vi "test-cubic-spline-00.vi"() -> (3 "Test Passed":bool)   [LabVIEW 2019]
uses:
  <vilib>/Rock Robotics/WPI/ThirdParty/JAS_Junk/TrajLib/POSEwCURVATURE.ctl
  <vilib>/Rock Robotics/WPI/ThirdParty/JAS_Junk/TrajLib/POSE2D.ctl
  <vilib>/Rock Robotics/WPI/ThirdParty/JAS_Junk/TrajLib/TRANSLATION2D.ctl
  <vilib>/Rock Robotics/WPI/ThirdParty/JAS_Junk/TrajLib/ROTATION2D.ctl
  <vilib>/Rock Robotics/WPI/ThirdParty/JAS_Junk/TrajLib/Rotation_CreateAngle.vi
  <vilib>/Rock Robotics/WPI/ThirdParty/JAS_Junk/TrajLib/Translation_Create.vi
  <vilib>/Rock Robotics/WPI/ThirdParty/JAS_Junk/TrajLib/Util_CalcDist.vi
  <vilib>/Rock Robotics/WPI/ThirdParty/JAS_Junk/TrajLib/Trajectory_Library.lvlib
panel:
  out "XY Graph":cluster{dbl[], dbl[]}(graph)
  out "All Interior \nwayPoints\nFound (True)":bool
  out "end rot = 0":dbl
  out "end y = 0":dbl
  out "end x = 0":dbl
  out "start rot = 0":dbl
  out "start y = 0":dbl
  out "start x = 0":dbl
  out "max dtheta < 0.0872":dbl
  out "max dy < 0.00127":dbl
  out "max dx  < 0.127":dbl
  out "Overall Error":errorcluster
  out "Elements":i32
  out "Create Spline Error":errorcluster
  out "SplinePoses\nWCurve":T1[](array[typedef]) {"POSE"."ROTATION"."SIN" format="%13.4f"; "POSE"."ROTATION"."COS" format="%13.4f"; "POSE"."ROTATION"."VALUE" format="%13.4f"; "POSE"."TRANSLATION"."Y" format="%14.3f"; "POSE"."TRANSLATION"."X" format="%14.3f"}
  out "Elapsed Time":dbl
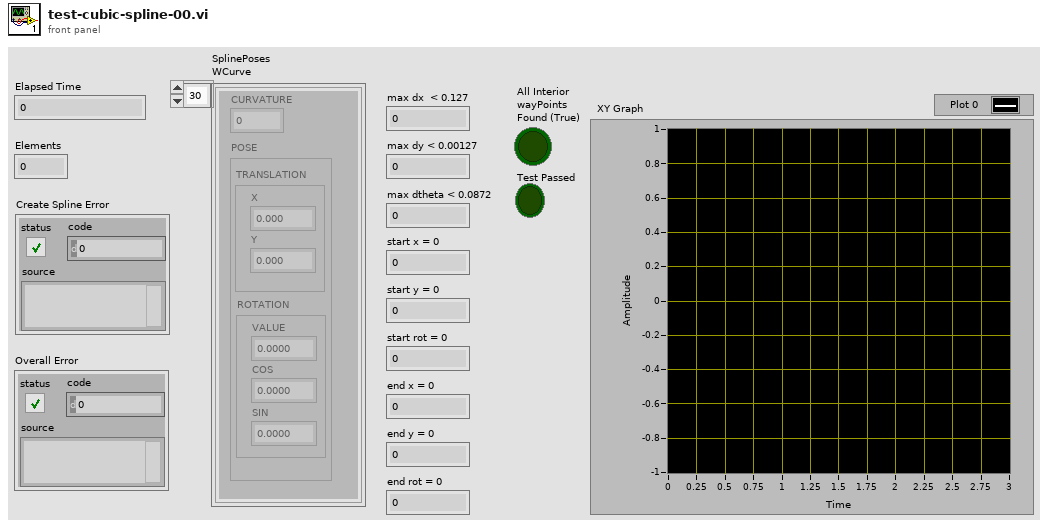
[diagram p1: front panel]
types:
  T1 = typedef "Trajectory_Library.lvlib/POSEwCURVATURE.ctl" = cluster{"CURVATURE":dbl, "POSE":T2}
  T2 = typedef "Trajectory_Library.lvlib/POSE2D.ctl" = cluster{"TRANSLATION":T3, "ROTATION":T4}
  T3 = typedef "Trajectory_Library.lvlib/TRANSLATION2D.ctl" = cluster{"X":dbl, "Y":dbl}
  T4 = typedef "Trajectory_Library.lvlib/ROTATION2D.ctl" = cluster{"VALUE":dbl, "COS":dbl, "SIN":dbl}
  T5 = typedef "Trajectory_Library.lvlib/SPLINE_CTRL_VECTOR.ctl" = cluster{"Xs":dbl[], "Ys":dbl[]}
  T6 = typedef "Trajectory_Library.lvlib/SPLINE.ctl" = cluster{"Degree":i32, "Coefficients":T7}
  T7 = typedef "NI_Matrix.lvlib/RealMatrix.ctl" = dbl[][]
  T8 = typedef "Trajectory_Library.lvlib/TWIST2D.ctl" = cluster{"dX":dbl, "dY":dbl, "dTHETA":dbl}
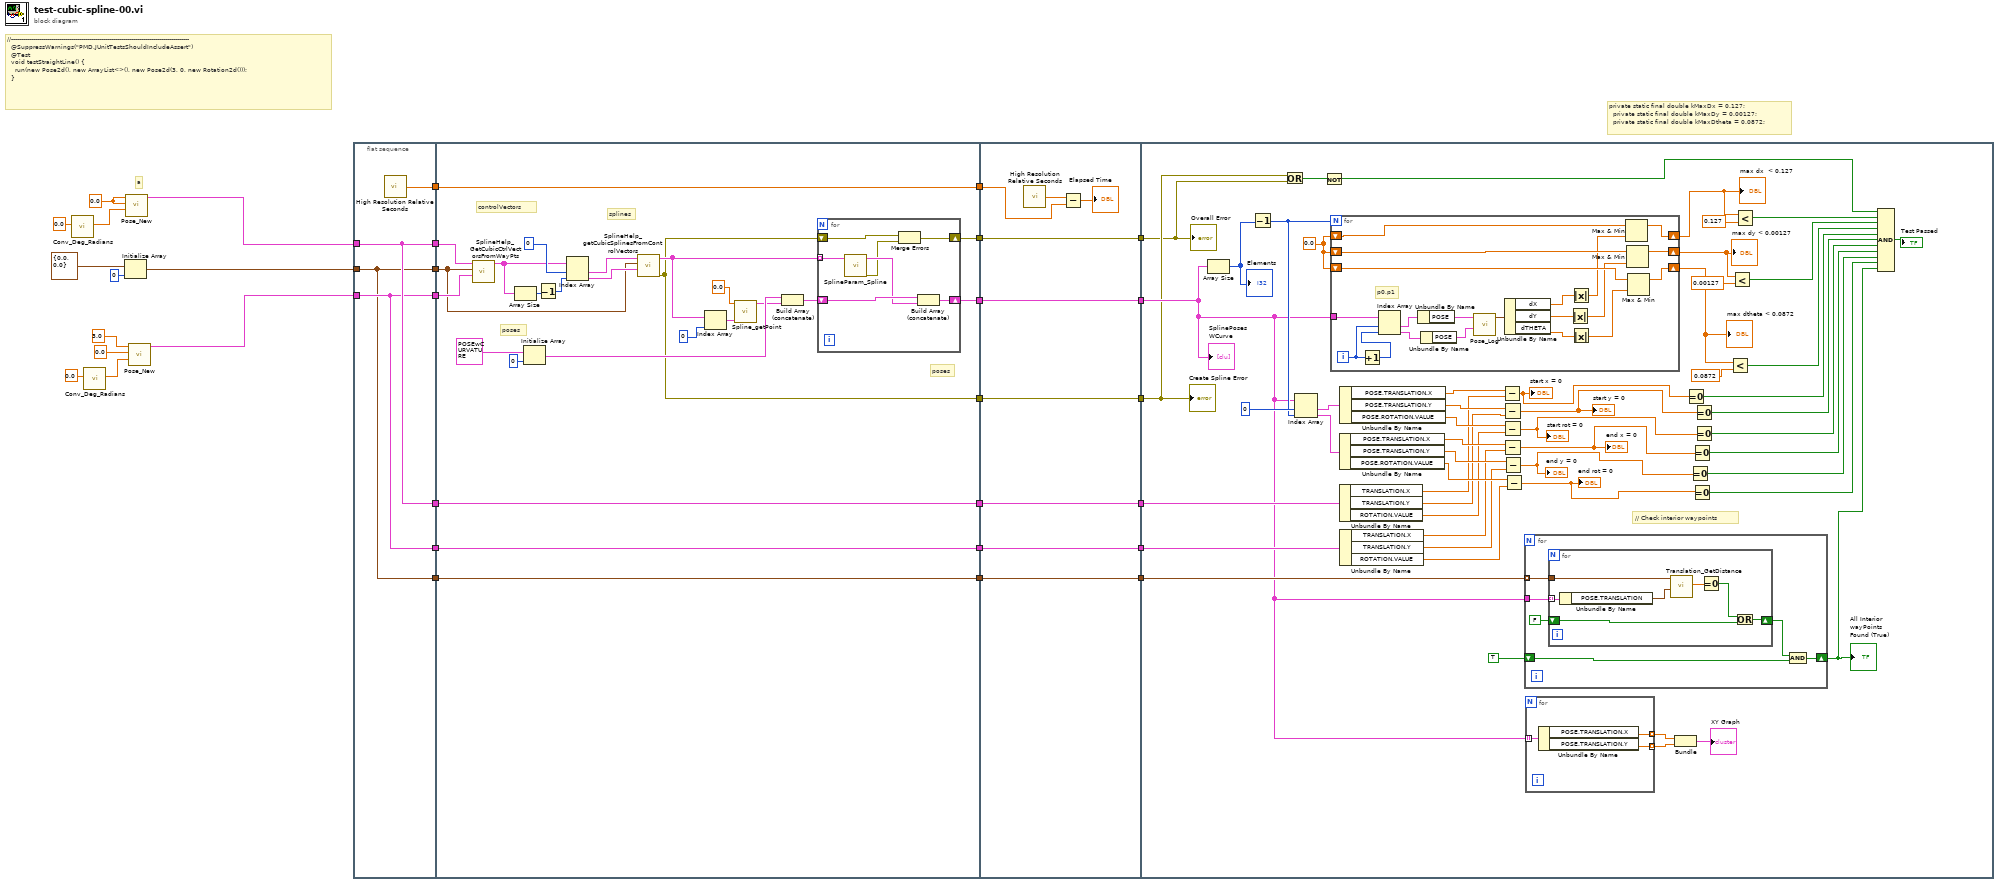
[diagram p0: block diagram]
diagram:
  w8 = 0.0 ("X")
  # "private static final double kMaxDx = 0.127;\n  private static final double kMaxDy = 0.00127;\n  private static final double kMaxDtheta = 0.0872;"
  # "a"
  # "//-----------------------------------------------------------------------------------------\n  @SuppressWarnings(\"PMD.JUnitTestsShouldIncludeAssert\")\n  @Test\n  void testStraightLine() {\n    run(new Pose2d(), new ArrayList<>(), new Pose2d(3, 0, new Rotation2d()));\n  }"
  n1 = call <vilib>:"Conv_Deg_Radians.vi"("Degress"=0.0) -> ("Radians"=w7:dbl)  [unwired: 10 in]
  n2 = call <vilib>:"Conv_Deg_Radians.vi"("Degress"=0.0) -> ("Radians"=w4:dbl)  [unwired: 10 in]
  n3 = Initialize Array(T3 {"X"=0.0, "Y"=0.0} ("TRANSLATION"), 0 ("dimension size")) -> (w1:T3[])
  n4 = call <vilib>:"Pose_New.vi"("Heading"=w7, "Y"=w8, "X"=w8) -> ("out POSe"=w30:T2)  [unwired: 8 in]
  n5 = call <vilib>:"Pose_New.vi"("Heading"=w4, "Y"=0.0, "X"=3.0) -> ("out POSe"=w27:T2)  [unwired: 8 in]
  n6 = flat-sequence {
    tunnel: w30 -> [w35]
    tunnel: [w35] -> w29
    tunnel: w1 -> [w33]
    tunnel: [w33] -> w28
    tunnel: w27 -> [w34]
    tunnel: [w34] -> w26
    tunnel: [w36] -> w25
    tunnel: [w35] -> w17
    tunnel: [w34] -> w14
    tunnel: [w33] -> w9
    tunnel: w29 -> [w61]
    tunnel: w28 -> [w53]
    tunnel: w26 -> [w60]
    tunnel: [w52] -> w24
    tunnel: w25 -> [w52]
    tunnel: [w42] -> w23
    tunnel: [w41] -> w21
    tunnel: [w40] -> w19
    tunnel: w17 -> [w39]
    tunnel: [w39] -> w16
    tunnel: w14 -> [w38]
    tunnel: [w38] -> w13
    tunnel: [w37] -> w10
    tunnel: w9 -> [w37]
    tunnel: w24 -> [w77]
    tunnel: w23 -> [w76]
    tunnel: [w76] -> w22
    tunnel: w21 -> [w75]
    tunnel: [w75] -> w20
    tunnel: w19 -> [w74]
    tunnel: [w74] -> w18
    tunnel: w16 -> [w71]
    tunnel: [w71] -> w15
    tunnel: w13 -> [w70]
    tunnel: [w70] -> w12
    tunnel: [w69] -> w11
    tunnel: w10 -> [w69]
    tunnel: w22 -> [w105]
    tunnel: w20 -> [w80]
    tunnel: w18 -> [w79]
    tunnel: w15 -> [w128]
    tunnel: w12 -> [w127]
    tunnel: w11 -> [w110]
    frame #0 {
      n7 = call <vilib>:"High Resolution Relative Seconds.vi"() -> ("relative seconds"=w36:dbl)
    }
    frame #1 {
      # "poses"
      # "poses"
      # "splines"
      # "controlVectors"
      n8 = call <vilib>:"SplineHelp_GetCubicCtrlVectorsFromWayPts.vi"("Enging POSE"=w60, "Interior WAYPOINTS"=w53, "Starting POSE"=w61) -> ("SplineControlVectors"=w57:T5[])  [unwired: 8 in]
      n9 = Array Size(array=w57) -> (size(s)=w58:i32)
      n10 = Initialize Array(T1 {"CURVATURE"=0.0, "POSE"={"TRANSLATION"={"X"=0.0, "Y"=0.0}, "ROTATION"={"VALUE"=0.0, "COS"=1.0, "SIN"=0.0}}} ("POSEwCURVATURE"), 0 ("dimension size")) -> (w46:T1[])
      n11 = Decrement(x=w58) -> (x-1=w56:i32)
      n12 = Index Array(array=w57, index #1=0 ("index"), index #2=w56) -> (element #1=w55:T5, element #2=w54:T5)
      n13 = call <vilib>:"SplineHelp_getCubicSplinesFromControlVectors.vi"("endCtrlVector"=w54, "InternalWaypoints"=w53, "startCtrlVector"=w55) -> ("error out"=w41:errorcluster, "splines"=w43:T6[])  [unwired: 3 in, 4 out]
      n14 = Index Array(array=w43, index=0) -> (element=w48:T6)
      n15 = call <vilib>:"Spline_getPoint.vi"("inputSPLINE"=w48, "Time"=0.0) -> ("POSEwCURVATURE"=w45:T1)  [unwired: 9 in]
      n16 = Build Array (concatenate)(w46, w45) -> (w44:T1[])
      n17 = for {
        shift-right: [w65] -> w42
        shift-left: w44 -> [w67]
        tunnel: w43 -> [w68] mode=indexing
        shift-right: [w63] -> w40
        shift-left: w41 -> [w64]
        n18 = call <vilib>:"SplineParam_Spline.vi"("inputSPLINE"=w68) -> ("error out"=w62:errorcluster, "outputPOSEwCURVATURE"=w66:T1[])  [unwired: 9 in]
        n19 = Merge Errors(w64, w62) -> (w63:errorcluster)
        n20 = Build Array (concatenate)(w67, w66) -> (w65:T1[])
      }
    }
    frame #2 {
      n21 = call <vilib>:"High Resolution Relative Seconds.vi"() -> ("relative seconds"=w72:dbl)
      n22 = Subtract(x=w72, y=w77) -> (x-y=→"Elapsed Time":dbl)
    }
    frame #3 {
      w129 = 0.0
      # "// Check interior waypoints"
      n23 = Array Size(array=w105) -> (size(s)=w130:i32)
      "Elements" <- w130
      n24 = Decrement(x=w130) -> (x-1=w125:i32)
      n25 = Or(x=w80, y=w79) -> (x .or. y?=w81:bool)
      n26 = Index Array(array=w105, index #1=0 ("index"), index #2=w125) -> (element #1=w124:T1, element #2=w123:T1)
      n27 = Not(x=w81) -> (.not. x?=w78:bool)
      n28 = for {
        N: w125 -> [_]
        tunnel: w105 -> [w164]
        shift-right: [w155] -> w102
        shift-left: w129 -> [w152]
        shift-right: [w153] -> w104
        shift-left: w129 -> [w150]
        shift-right: [w154] -> w103
        shift-left: w129 -> [w151]
        i -> [w166]
        # "p0,p1"
        n29 = Increment(x=w166) -> (x+1=w165:i32)
        n30 = Index Array(array=w164, index #1=w166, index #2=w165) -> (element #1=w163:T1, element #2=w162:T1)
        n31 = Unbundle By Name(w163) -> ("POSE"=w161:T2)
        n32 = Unbundle By Name(w162) -> ("POSE"=w160:T2)
        n33 = call <vilib>:"Pose_Log.vi"("end POSE"=w160, "in POSE"=w161) -> ("out TWIST"=w159:T8)  [unwired: 9 in]
        n34 = Unbundle By Name(w159) -> ("dX"=w156:dbl, "dY"=w157:dbl, "dTHETA"=w158:dbl)
        n35 = Absolute Value(x=w157) -> (abs(x)=w148:dbl)
        n36 = Absolute Value(x=w156) -> (abs(x)=w149:dbl)
        n37 = Absolute Value(x=w158) -> (abs(x)=w147:dbl)
        n38 = Max & Min(x=w152, y=w149) -> (max(x,y)=w155:dbl)  [unwired: 1 out]
        n39 = Max & Min(x=w151, y=w148) -> (max(x,y)=w154:dbl)  [unwired: 1 out]
        n40 = Max & Min(x=w150, y=w147) -> (max(x,y)=w153:dbl)  [unwired: 1 out]
      }
      "max dx  < 0.127" <- w102
      "max dy < 0.00127" <- w103
      "max dtheta < 0.0872" <- w104
      n41 = Unbundle By Name(w123) -> ("POSE.TRANSLATION.X"=w119:dbl, "POSE.TRANSLATION.Y"=w118:dbl, "POSE.ROTATION.VALUE"=w117:dbl)
      n42 = Unbundle By Name(w128) -> ("TRANSLATION.X"=w116:dbl, "TRANSLATION.Y"=w115:dbl, "ROTATION.VALUE"=w114:dbl)
      n43 = Unbundle By Name(w124) -> ("POSE.TRANSLATION.X"=w122:dbl, "POSE.TRANSLATION.Y"=w121:dbl, "POSE.ROTATION.VALUE"=w120:dbl)
      n44 = Unbundle By Name(w127) -> ("TRANSLATION.X"=w113:dbl, "TRANSLATION.Y"=w112:dbl, "ROTATION.VALUE"=w111:dbl)
      n45 = Subtract(x=w122, y=w116) -> (x-y=w95:dbl)
      "start x = 0" <- w95
      n46 = Subtract(x=w121, y=w115) -> (x-y=w94:dbl)
      "start y = 0" <- w94
      n47 = Subtract(x=w120, y=w114) -> (x-y=w93:dbl)
      "start rot = 0" <- w93
      n48 = Subtract(x=w119, y=w113) -> (x-y=w92:dbl)
      "end x = 0" <- w92
      n49 = Subtract(x=w118, y=w112) -> (x-y=w91:dbl)
      "end y = 0" <- w91
      n50 = Subtract(x=w117, y=w111) -> (x-y=w90:dbl)
      "end rot = 0" <- w90
      n51 = for {
        tunnel: w110 -> [w134] mode=indexing
        tunnel: w105 -> [w139]
        shift-right: [w138] -> w83
        shift-left: TRUE -> [w137]
        n52 = for {
          tunnel: w139 -> [w143] mode=indexing
          shift-right: [w146] -> w135
          shift-left: FALSE -> [w145]
          tunnel: w134 -> [w144]
          n53 = Unbundle By Name(w143) -> ("POSE.TRANSLATION"=w142:T3)
          n54 = call <vilib>:"Translation_GetDistance.vi"("other Translation"=w142, "In Translation"=w144) -> ("Distance"=w141:dbl)  [unwired: 9 in]
          n55 = Equal To 0?(x=w141) -> (x = 0?=w140:bool)
          n56 = Or(x=w140, y=w145) -> (x .or. y?=w146:bool)
        }
        n57 = And(x=w135, y=w137) -> (x .and. y?=w138:bool)
      }
      "All Interior \nwayPoints\nFound (True)" <- w83
      n58 = for {
        tunnel: [w133] -> w108 mode=indexing
        tunnel: [w132] -> w107 mode=indexing
        tunnel: w105 -> [w131] mode=indexing
        n59 = Unbundle By Name(w131) -> ("POSE.TRANSLATION.X"=w133:dbl, "POSE.TRANSLATION.Y"=w132:dbl)
      }
      n60 = Bundle(w108, w107) -> (→"XY Graph":cluster{dbl[], dbl[]})  [unwired: 1 in]
      n61 = Equal To 0?(x=w95) -> (x = 0?=w89:bool)
      n62 = Equal To 0?(x=w91) -> (x = 0?=w85:bool)
      n63 = Equal To 0?(x=w92) -> (x = 0?=w86:bool)
      n64 = Equal To 0?(x=w90) -> (x = 0?=w84:bool)
      n65 = Equal To 0?(x=w94) -> (x = 0?=w88:bool)
      n66 = Equal To 0?(x=w93) -> (x = 0?=w87:bool)
      n67 = Less?(x=w104, y=0.0872) -> (x < y?=w96:bool)
      n68 = Less?(x=w103, y=0.00127) -> (x < y?=w97:bool)
      n69 = Less?(x=w102, y=0.127) -> (x < y?=w98:bool)
      n70 = Compound Arithmetic op=AND(w78, w98, w97, w96, w89, w88, w87, w86, w85, w84, w83) -> (→"Test Passed":bool)
      "SplinePoses\nWCurve" <- w105
      "Create Spline Error" <- w80
      "Overall Error" <- w79
    }
  }
